vi "RSZVB Set Power Coeficients Default.vi"(8 "error in (no error)":errorcluster {"code" format="%.0x"}, 10 "Default Coeficients (Off)":bool, 11 "VISA session":refnum<visa-resource-name>) -> (0 "error out":errorcluster {"code" format="%.0x"}, 3 "dup VISA session":refnum<visa-resource-name>)   [LabVIEW 2011]
doc: "Enables or disables default power coefficients for frequency converters R&S ZVA-ZxxxE. \n\nNotes:\n\n(1) This command is available for frequency converters with electronic attenuators R&S ZVA-ZxxxE.\n\nRemote-control command(s):\n[SENSe<Ch>:]FREQuency:CONVersion:DEVice:PCOefficient<Port>:DEFault"
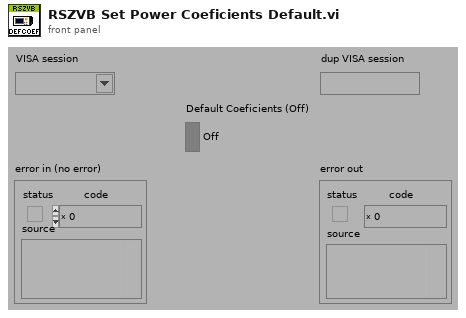
[diagram p1: front panel]
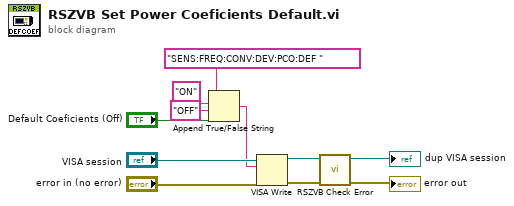
[diagram p0: block diagram]
diagram:
  n1 = Append True/False String(1:"Default Coeficients (Off)", 2:"OFF" ("false string"), 3:"ON" ("true string"), 4:"SENS:FREQ:CONV:DEV:PCO:DEF " ("string (\"\")")) -> (0:w5:string)
  n2 = VISA Write(VISA resource name="VISA session", write buffer=w5, error in (no error)="error in (no error)") -> (VISA resource name out=w3:refnum<visa-resource-name>, error out=w4:errorcluster)  [unwired: 1 out]
  n3 = call "RSZVB Check Error.vi"("error in (no error)"=w4, "VISA session"=w3) -> ("error out"=→"error out":errorcluster, "dup VISA session"=→"dup VISA session":refnum<visa-resource-name>)  [unwired: 8 in]
